vi "Global 1.vi"() -> ()   [LabVIEW 2018]
panel:
  out "Handle":u64
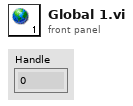
[diagram p1: front panel]
diagram:
